vi "MM6.LoadObjs.vi"(0 "i ref in":refnum<vi>, 3 "ms timeout (10000)":i32=10000, 5 "error in (no error)":errorcluster) -> (14 "i ref out":refnum<vi>, 17 "timed out":bool, 19 "error out":errorcluster)   [LabVIEW 2014, in "MM6.lvlib"]
doc: "This method loads all requested device objects by looking them up in the UsedObjs attribute table."
uses:
  MM6.lvlib
  CS_Core/CSSystem/CoreDefs/CoreDefs.error_type.ctl
  CS_Core/CSSystem/CoreDefs/CoreDefs.error_severity.ctl
  CS_Core/CSSystem/CoreLib/CoreLib.string 2 byte array.vi
  CS_Core/BaseProcess/BaseProcess.lvlib
  CS_Core/CSSystem/CoreLib/CoreLib.lvlib
  CS_Core/CSSystem/CSSystemLib/CSSystemLib.lvlib
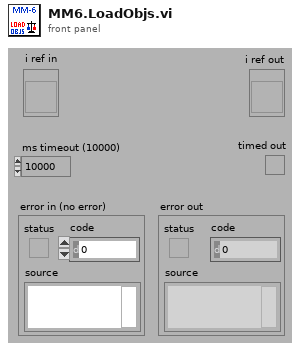
[diagram p1: front panel]
types:
  T1 = typedef "CoreDefs.error_severity.ctl" = enum16{"undefined", "information", "warning", "error", "fatal"}
  T2 = typedef "CoreDefs.error_type.ctl" = enum16{"no error", "can't load process", "can't unload process", "process does not exist", "can't install process", "can't remove process", "unknown function", "time out", "can't execute function", "duplicate queue name", "super not found", "caller queue invalid", "can't ping process", "unknown error", "VISA Error", "VISA timeout", "GPIB timeout", "GPIB error", "communication error", "data type mismatch", "can't read data from OPC server", "can't write data to OPC server", "OET error", "function not implemented", "process already exists", "invalid Shared Variable name", "error writing Shared Variable", "error reading Shared Variable", "invalid client name", "corrupt database", "unknown class", "call not authorized", "parameter out of range", "OET timeout: can't get data to modify", "invalid queue name", "requested operation incompatible with current state", "event undefined", "event disabled", "state undefined", "caller is not a friend", "EventBuilder: bad eventID", "EventBuilder: no DAQ devices", "a thread must not stop itself", "UNUSED ELEMENT4", "DiscArchiver: eventData incomplete", "DiscArchiver: eventData does not belong to run", "DiscArchiver: can't open file", "DiscArchiver: can't write to file", "DiscArchiver: available disc space low", "can't acquire semaphore", "error reading data from database", "notifier object is not existing", "can't register process", "can't unregister process", "illegal event type", "object disabled", "object already exists", "can't change state", "Instrument not found", "no connection to remote node", "invalid reference", "N/A", "UNUSED ELEMENT 1", "element not found", "illegal TCP/IP connection detected", "object does not exist", "invalid access ID", "unknown CS system", "invalid privilige", "unsupported data type", "unsupported server type", "IO server already exists", "Shared Variable already exists"}
  T3 = typedef "MM6.lvlib/MM6.i attribute.ctl" = cluster{"ConfigData":T4, "UsedObjs":string[], "ActScanStep":i32[], "AbortRequest":bool, "StopRequest":bool, "# cycles":i32, "Connected":bool, "MMStatus":T19, "# data":i32, "DIMServices":cluster{"MM6StatusString":string, "MM6StatusID":i32, "discArchiver":string, "discArchiverID":i32, "eventBuilder":string, "eventBuilderID":i32, "GUIIDString":string, "GUIIDStringID":i32}, "dataFile":string, "ExtraDataSets":T20, "PGRunning":T21}
  T4 = typedef "LEBITDefs.lvlib/LEBITDefs.ConfigData.ctl" = cluster{"GenConfig":T5, "Configs":T7[]}
  T5 = typedef "LEBITDefs.lvlib/LEBITDefs.GenConfig.ctl" = cluster{"Mode":i32, "Logs":T6[]}
  T6 = typedef "LEBITDefs.lvlib/LEBITDefs.Log.ctl" = cluster{"Name":string, "FctName":string, "Special":string}
  T7 = typedef "LEBITDefs.lvlib/LEBITDefs.OneConfig.ctl" = cluster{"MCA":T8, "Timing":T9, "Scans":T12[], "FreqDevs":T13[], "CleanDev":T14, "NrCycles":i32, "Specials":T16[], "Delays":T17[], "DAC":T18}
  T8 = typedef "LEBITDefs.lvlib/LEBITDefs.MCA.ctl" = cluster{"Name":string, "Address":string, "NrChannels":i32, "Gate":i32, "NrPipse":i32}
  T9 = typedef "LEBITDefs.lvlib/LEBITDefs.Timing.ctl" = cluster{"TimeTables":cluster{"TimeTable":T10}[], "Memories":T11[], "ScanX":string, "ScanY":string}
  T10 = typedef "LEBITDefs.lvlib/LEBITDefs.Timetable.ctl" = dbl[]
  T11 = typedef "LEBITDefs.lvlib/LEBITDefs.Memory.ctl" = cluster{"Device":string, "ExtTrig":bool, "TT2Use":i32, "PatternTable":string[]}
  T12 = typedef "LEBITDefs.lvlib/LEBITDefs.ScanDev.ctl" = cluster{"Name":string, "FctName":string, "Values":dbl[], "NrScanVals":i32, "Special":string}
  T13 = typedef "LEBITDefs.lvlib/LEBITDefs.FreqDev.ctl" = cluster{"Name":string, "Amp":dbl, "CenterFreq":dbl, "Time":dbl}
  T14 = typedef "LEBITDefs.lvlib/LEBITDefs.CleanDev.ctl" = cluster{"Name":string, "CleanData":T15[]}
  T15 = typedef "LEBITDefs.lvlib/LEBITDefs.CleanDataType.ctl" = cluster{"Amp":dbl, "Center":dbl, "Plus":dbl, "Minus":dbl, "Time":dbl}
  T16 = typedef "LEBITDefs.lvlib/LEBITDefs.Special.ctl" = cluster{"Name":string, "FctName":string, "VerySpecial":string, "Data":dbl}
  T17 = typedef "LEBITDefs.lvlib/LEBITDefs.Delay.ctl" = cluster{"Name":string, "Delay":dbl}
  T18 = typedef "LEBITDefs.lvlib/LEBITDefs.DAC.ctl" = cluster{"Name":string, "Step1":i32, "Step2":i32}
  T19 = typedef "MM6.lvlib/MM6.status.ctl" = enum16{"loaded", "load_error", "config", "config_error", "init", "init_error", "data_reset", "data_reset_error", "running", "start_error", "run_error", "abort_requested", "aborted", "stop_requested", "stopped", "stop_error", "Connected", "NOTConnected"}
  T20 = typedef "LEBITDefs.lvlib/LEBITDefs.ExtraData.ctl" = cluster{"Ions":cluster{"ExcitIonMass":string, "ExcitIonCharge":i32, "CleanIons":cluster{"CleanIonMass":string, "CleanIonCharge":i32}[]}, "TimingDescription":cluster{"TimeTableDescription":cluster{"Times":string[]}[], "PatternTableDescription":cluster{"Pattern":string[]}[]}, "ScanUnits":string[]}[]
  T21 = typedef "PPG_ABC.lvlib/PPG_ABC.PG_Running.ctl" = i32
  T22 = typedef "CoreDefs.rawDataType.ctl" = i8[]
  T23 = typedef "CoreDefs.call_type.ctl" = cluster{"Object":string, "Selector":string, "CallType":enum16{"simple", "synchronous", "asynchronous"}, "Async Object":string, "Async Selector":string, "Data Descriptor":T24, "Data":T22, "Error #":i32, "Expire":u32}
  T24 = typedef "BaseProcess.lvlib/BaseProcess.descriptor string definition.ctl" = string
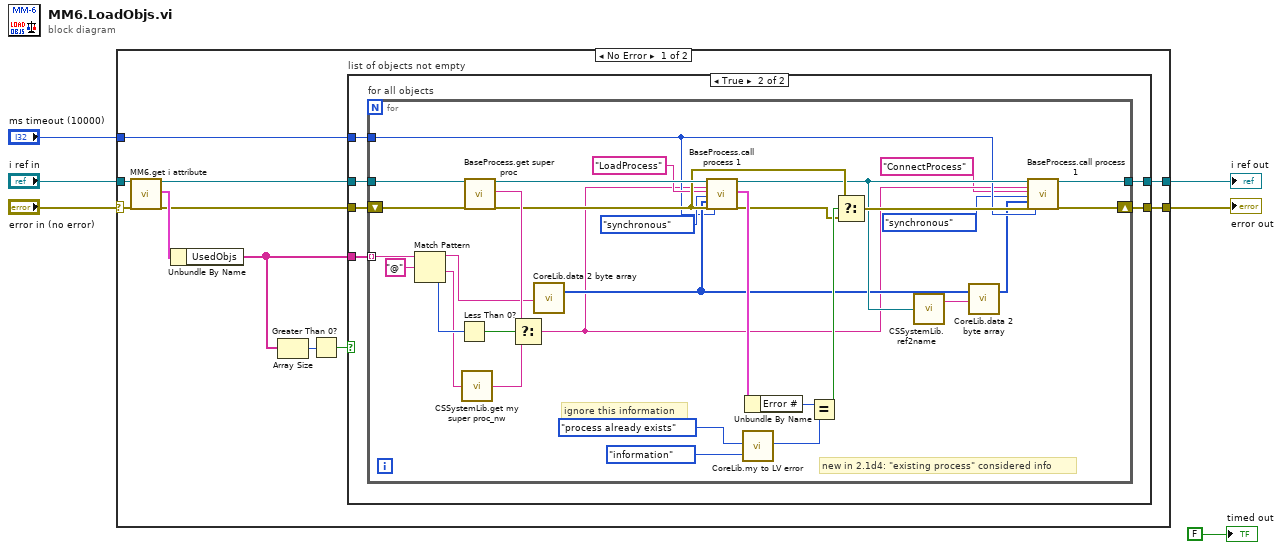
[diagram p0: block diagram]
diagram:
  n1 = case shown="No Error" "error in (no error)" {
    selector: "error in (no error)" -> [w7 w58]
    tunnel: "i ref in" -> [w17 w59]
    tunnel: [w14 w59] -> w5
    tunnel: [w12 w58] -> w3
    tunnel: "ms timeout (10000)" -> [w8 _]
    frame No Error {
      n2 = call "MM6.get i attribute.vi"("i ref in"=w17, "error in (no error)"=w7) -> ("i ref out"=w15:refnum<vi>, "i attribute"=w16:T3, "error out"=w13:errorcluster)  [unwired: 15 in]
      n3 = Unbundle By Name(w16) -> ("UsedObjs"=w11:string[])
      n4 = Array Size(array=w11) -> (size(s)=w9:i32)
      n5 = Greater Than 0?(x=w9) -> (x > 0?=w10:bool)
      n6 = case "list of objects not empty" shown="True" w10 {
        tunnel: w11 -> [_ w25]
        tunnel: w15 -> [w19 w24]
        tunnel: [w19 w23] -> w14
        tunnel: w13 -> [w18 w22]
        tunnel: [w18 w21] -> w12
        tunnel: w8 -> [_ w20]
        frame False {
        }
        frame True {
          n7 = for "for all objects" {
            tunnel: w25 -> [w57] mode=indexing
            tunnel: w24 -> [w54]
            tunnel: [w50] -> w23
            shift-right: [w41] -> w21
            shift-left: w22 -> [w49]
            tunnel: w20 -> [w30]
            # "new in 2.1d4: \"existing process\" considered info"
            # "ignore this information"
            n8 = Match Pattern(string=w57, regular expression="@") -> (before substring=w36:string, after substring=w35:string, offset past match=w55:i32)  [unwired: 1 in, 1 out]
            n9 = Less Than 0?(x=w55) -> (x < 0?=w52:bool)
            n10 = call "CSSystemLib.get my super proc_nw.vi"("systemID"=w35) -> ("superProcName"=w34:string)
            n11 = call "BaseProcess.get super proc.vi"("i ref in"=w54, "error in (no error)"=w49) -> ("i ref out"=w53:refnum<vi>, "SuperProc"=w51:string, "error out"=w42:errorcluster)  [unwired: 15 in]
            n12 = Select(t=w51, s=w52, f=w34) -> (s? t:f=w29:string)
            n13 = call-poly "CoreLib.data 2 byte array.vi"("string"=w36) -> ("byteArray out"=w32:T22)  [unwired: 18 in]
            n14 = call "BaseProcess.call process 1.vi"("i ref in"=w53, "Object"=w29, "Selector"="LoadProcess", "CallType"=enum16{"simple", "synchronous", "asynchronous"}."synchronous", "Data"=w32, "error in (no error)"=w42, "timeout (ms)"=w30) -> ("i ref out"=w39:refnum<vi>, "call cluster out"=w48:T23, "error out"=w43:errorcluster)  [unwired: 10 in]
            n15 = call "CoreLib.my to LV error.vi"("ErrorTypes"=CoreDefs.error_type."process already exists", "severityLevel"=CoreDefs.error_severity."information") -> ("LV error code"=w45:i32)  [unwired: 16 in, 1 out]
            n16 = Unbundle By Name(w48) -> ("Error #"=w47:i32)
            n17 = Equal?(x=w47, y=w45) -> (x = y?=w44:bool)
            n18 = Select(t=w42, s=w44, f=w43) -> (s? t:f=w40:errorcluster)
            n19 = call "CSSystemLib.ref2name.vi"("obj refnum"=w39) -> ("name"=w37:string)
            n20 = call-poly "CoreLib.data 2 byte array.vi"("byteArray"=w32, "string"=w37) -> ("byteArray out"=w26:T22)  [unwired: 17 in]
            n21 = call "BaseProcess.call process 1.vi"("i ref in"=w39, "Object"=w29, "Selector"="ConnectProcess", "CallType"=enum16{"simple", "synchronous", "asynchronous"}."synchronous", "Data"=w26, "error in (no error)"=w40, "timeout (ms)"=w30) -> ("i ref out"=w50:refnum<vi>, "error out"=w41:errorcluster)  [unwired: 10 in, 1 out]
          }
        }
      }
    }
    frame Error {
    }
  }
  "error out" <- w3
  "i ref out" <- w5
  "timed out" <- FALSE ("timed out")
